vi "mcc_usb202_read.vi"(6 "error in":errorcluster, 11 "task in":refnum<k24>) -> (0 "status":bool=TRUE, 1 "V1":dbl, 2 "V0":dbl, 3 "task out":refnum<k24>, 4 "error out":errorcluster={"status"=TRUE, "code"=10023, "source"="ULx Create Channel (AI-Voltage-Basic).vi:5780001<ERR>\nMeasurements: Channel not specified."})   [LabVIEW 2019]
uses:
  C:/Program Files/National Instruments/LabVIEW 2019/vi.lib/ULx/ULx_LV.dll
  Program Files/National Instruments/LabVIEW 2019/vi.lib/ULx/ULx_LV.dll
  <vilib>/ULx/Read.llb/ULx Read (Analog 1D DBL NChan 1Samp).vi
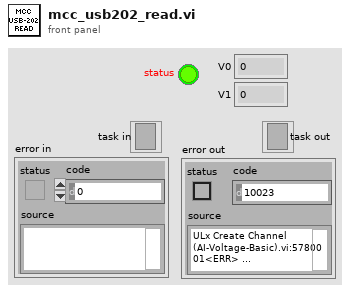
[diagram p1: front panel]
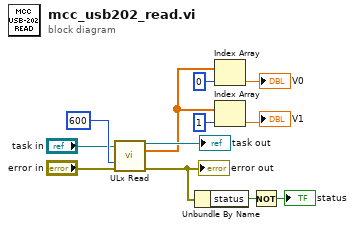
[diagram p0: block diagram]
diagram:
  n1 = call-poly <vilib>:"ULx Read.vi"("task in"="task in", "timeout"=600, "error in"="error in") -> ("task out"=→"task out":refnum<k24>, "data"=w3:dbl[], "error out"=w8:errorcluster)  [unwired: 10 in]
  "error out" <- w8
  n2 = Unbundle By Name(w8) -> ("status"=w7:bool)
  n3 = Index Array(array=w3, index=0) -> (element=→"V0":dbl)
  n4 = Index Array(array=w3, index=1) -> (element=→"V1":dbl)
  n5 = Not(x=w7) -> (.not. x?=→"status":bool)
